vi "remote delay.vi"(7 "second":dbl, 8 "dt(s)":dbl, 9 "i":i32) -> (1 "i out":i32, 2 "finish?":bool)   [LabVIEW 2019]
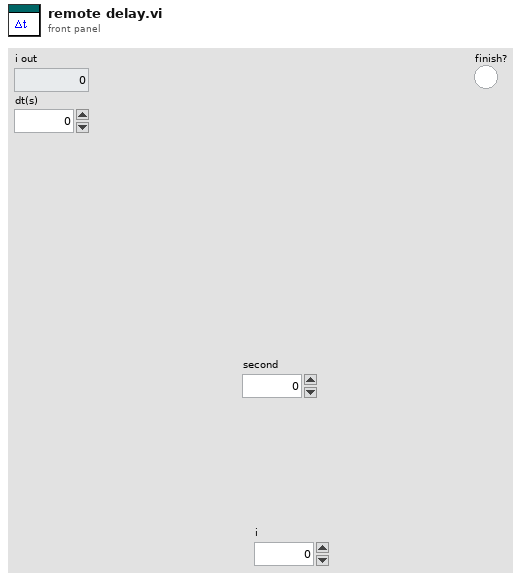
[diagram p1: front panel]
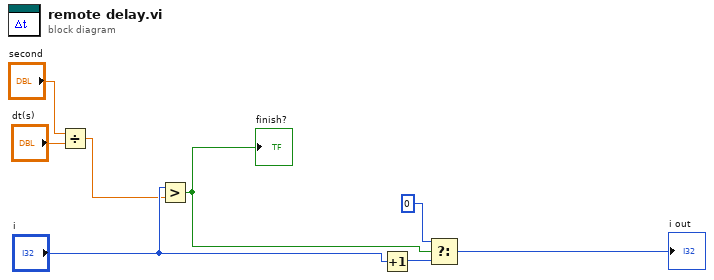
[diagram p0: block diagram]
diagram:
  n1 = Divide(x="second", y="dt(s)") -> (x/y=w3:dbl)
  n2 = Greater?(x="i", y=w3) -> (0:w2:bool)
  "finish?" <- w2
  n3 = Increment(x="i") -> (x+1=w6:i32)
  n4 = Select(t=0, s=w2, f=w6) -> (s? t:f=→"i out":i32)
